vi "setPulsatorSpeed.vi"(8 "comms":T2, 10 "speed data":variant, 11 "Queues":T1) -> ()   [LabVIEW 2018]
uses:
  type defs/comms loop data.ctl
  ICL-LabVIEW_General/Incident logger/Incident logger.lvclass
  <vilib>/Modbus/master/Modbus Master.lvclass
  type defs/Queues.ctl
  <vilib>/Utility/error.llb/Error Cluster From Error Code.vi
  ICL-LabVIEW_General/Pulser Controller/AKD MODBUS commands/set velocity.vi
  ICL-LabVIEW_General/Pulser Controller/AKD MODBUS commands/stop drive.vi
  ICL-LabVIEW_General/Pulser Controller/AKD MODBUS commands/start drive.vi
  <vilib>/ErrorRing/Error Ring.xnode
  ICL-LabVIEW_General/Pulser Controller/Pulser controller commands library.lvlib
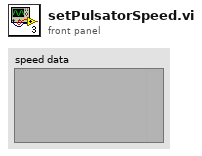
[diagram p1: front panel]
types:
  T1 = typedef "Queues.ctl" = cluster{"messageHandler":refnum<queue>, "comms":refnum<queue>, "dataStream":refnum<queue>, "dataProcessor":refnum<queue>, "fileIO":refnum<queue>, "userInterface":refnum<queue>, "errors":refnum<queue>, "customCompressor":refnum<queue>}
  T2 = typedef "comms loop data.ctl" = cluster{"params":cluster{"commandStream":cluster{"reader name":string, "writer name":string, "stream buffer size":i32}, "errorStream":cluster{"reader name":string, "writer name":string, "stream buffer size":i32}, "RT IP address":string, "pulserControllerIP":string}, "vars":cluster{"commandStream":refnum<k21>, "Incident logger":refnum<class "Incident logger.lvclass">, "check error scheduled message":u32, "errorStream":refnum<k21>, "watchdogScheduleID":u32, "pulsator":cluster{"pulser connection":refnum<class "Modbus Master.lvclass">, "pulserConnected":bool, "pulsatorScheduleID":u32, "pulserRunning":bool, "pulsatorRetries":u8}}}
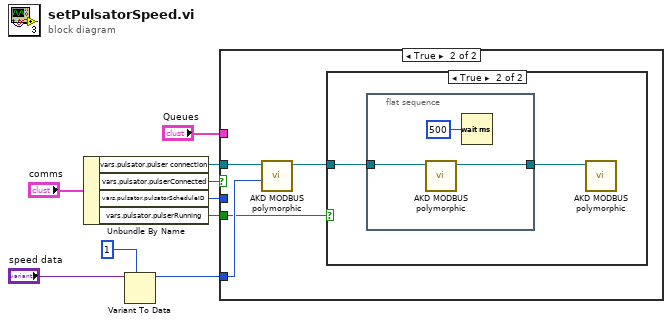
[diagram p0: block diagram]
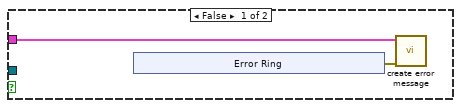
[diagram p2: hidden frame]
diagram:
  n1 = Unbundle By Name("comms") -> ("vars.pulsator.pulser connection"=w6:refnum<class "Modbus Master.lvclass">, "vars.pulsator.pulserConnected"=w8:bool, "vars.pulsator.pulsatorScheduleID"=w7:u32, "vars.pulsator.pulserRunning"=w1:bool)
  n2 = Variant To Data(type=u32 1 ("Velocity (RPM)"), Variant="speed data") -> (data=w3:u32)  [unwired: 1 in, 1 out]
  n3 = case shown="True" w8 {
    tunnel: w7 -> [_ _]
    tunnel: w6 -> [_ w20]
    tunnel: "Queues" -> [w11 _]
    tunnel: w3 -> [_ w19]
    tunnel: w1 -> [_ w18]
    frame False {
      n4 = xnode "Error Ring"() -> ("error out"=w10:errorcluster)
      n5 = call "create error message.vi"("error in (no error)"=w10, "queues"=w11) -> ()  [unwired: 10 in]
    }
    frame True {
      n6 = call-poly "AKD MODBUS polymorphic.vi"("Velocity (RPM)"=w19, "Modbus Master in"=w20) -> ("Modbus Master out"=w17:refnum<class "Modbus Master.lvclass">)  [unwired: 9 in]
      n7 = case shown="True" w18 {
        tunnel: w17 -> [_ w22]
        frame False {
        }
        frame True {
          n8 = flat-sequence {
            tunnel: w22 -> [w25]
            tunnel: [w23] -> w21
            frame #0 {
              n9 = call-poly "AKD MODBUS polymorphic.vi"("Modbus Master in"=w25) -> ("Modbus Master out"=w23:refnum<class "Modbus Master.lvclass">)  [unwired: 10 in]
              n10 = Wait (ms)(milliseconds to wait=u32 500) -> ()  [unwired: 1 out]
            }
          }
          n11 = call-poly "AKD MODBUS polymorphic.vi"("Modbus Master in"=w21) -> ()  [unwired: 10 in, 1 out]
        }
      }
    }
  }
